vi "SN Gen.vi"(6 "Last MFG Date":string, 8 "error in (no error)":errorcluster, 9 "Date and Shift In":string, 10 "SN In":i64, 11 "PN In":string) -> (0 "error out":errorcluster, 1 "Full SN Out":string, 2 "SN":string, 3 "SN Out":i64)   [LabVIEW 2018]
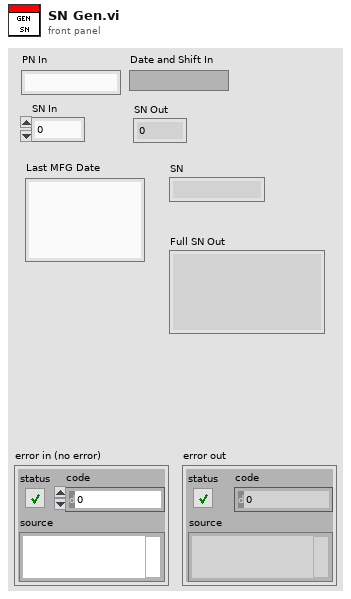
[diagram p1: front panel]
types:
  T1 = typedef "LVDateTimeRec.ctl" = cluster{"fractional second":dbl, "second":i32, "minute":i32, "hour":i32, "day of month":i32, "month":i32, "year":i32, "day of week":i32, "day of year":i32, "DST":i32}
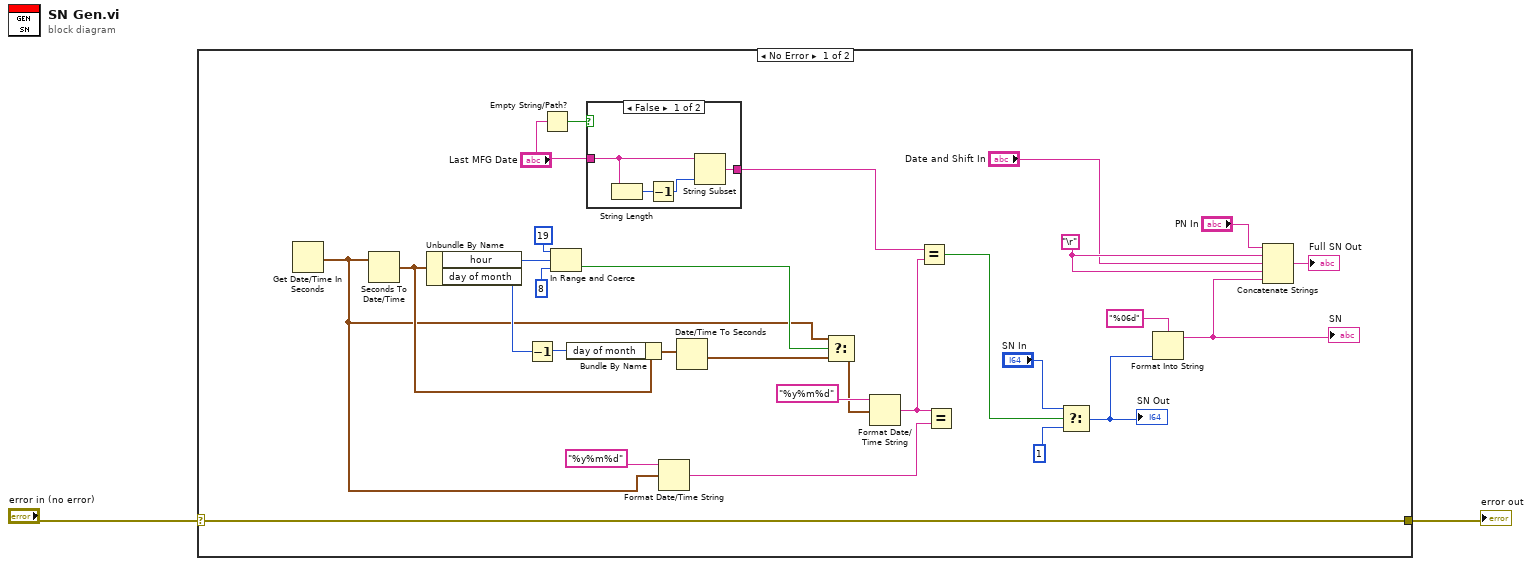
[diagram p0: block diagram]
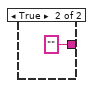
[diagram p2: hidden frame]
diagram:
  n1 = case shown="No Error" "error in (no error)" {
    selector: "error in (no error)" -> [w17 w37]
    tunnel: [w17 w37] -> w1
    frame No Error {
      w13 = "\r"
      n2 = Get Date/Time In Seconds() -> (seconds since 1Jan1904=w11:timestamp)
      n3 = Seconds To Date/Time(time stamp (now)=w11) -> (date time rec=w21:T1)  [unwired: 1 in]
      n4 = Unbundle By Name(w21) -> ("hour"=w27:i32, "day of month"=w25:i32)
      n5 = Decrement(x=w25) -> (x-1=w28:i32)
      n6 = Empty String/Path?(string/path="Last MFG Date") -> (empty?=w3:bool)
      n7 = In Range and Coerce(upper limit=i16 19, x=w27, lower limit=i16 8 ("upper limit")) -> (In Range?=w24:bool)  [unwired: 1 out]
      n8 = Bundle By Name(cluster=w21, "day of month"=w28) -> (w26:T1)
      n9 = case shown="False" w3 {
        tunnel: "Last MFG Date" -> [w35 _]
        tunnel: [w32 "" ("Last MFG Date")] -> w7
        frame False {
          n10 = String Length(string=w35) -> (length=w34:i32)
          n11 = Decrement(x=w34) -> (x-1=w33:i32)
          n12 = String Subset(string=w35, length (rest)=w33) -> (substring=w32:string)  [unwired: 1 in]
        }
        frame True {
        }
      }
      n13 = Format Date/Time String(time format string (%c)="%y%m%d", seconds (now)=w11) -> (date/time string=w10:string)  [unwired: 1 in]
      n14 = Date/Time To Seconds(2:w26) -> (0:w23:timestamp)  [unwired: 1 in]
      n15 = Select(t=w11, s=w24, f=w23) -> (s? t:f=w22:timestamp)
      n16 = Format Date/Time String(time format string (%c)="%y%m%d", seconds (now)=w22) -> (date/time string=w6:string)  [unwired: 1 in]
      n17 = Equal?(x=w7, y=w6) -> (x = y?=w5:bool)
      n18 = Equal?(x=w6, y=w10) -> ()  [unwired: 1 out]
      n19 = Select(t="SN In", s=w5, f=1) -> (s? t:f=w14:i64)
      "SN Out" <- w14
      n20 = Format Into String(format string="%06d", w14) -> (resulting string=w9:string)  [unwired: 2 in, 1 out]
      "SN" <- w9
      n21 = Concatenate Strings("PN In", w13, "Date and Shift In", w13, w9) -> (→"Full SN Out":string)
    }
    frame Error {
    }
  }
  "error out" <- w1
